vi "Send Message to Notebook.vi"(2 "Notebook Queue":refnum<queue>, 4 "Message":string, 5 "Error In":errorcluster, 9 "Text Formatting":T1={"Font"="Default", "Text Color"=enum."Unchanged", "Text Background Color"=enum."Unchanged", "Text Style"=enum."Regular", "Font Size (Points)"=-1.0, "Text Alignment"=0} {"Text Alignment" items=["Left", "Right", "Center"]}) -> (19 "Error Out":errorcluster)   [LabVIEW 2019, in "Notebook.lvlib"]
uses:
  Notebook.lvlib
  Notebook Action Q Element.ctl
  Notebook Action List.ctl
  Rich Text Box/Text Formatting.ctl
  Rich Text Box/Text Colors.ctl
  Rich Text Box/Formatted Text.ctl
  Rich Text Box/Rich Text Box.lvlib
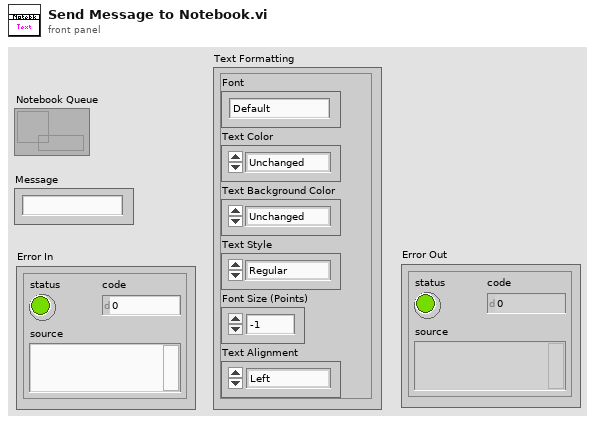
[diagram p1: front panel]
types:
  T1 = typedef "Rich Text Box.lvlib/Text Formatting.ctl" = cluster{"Font":string, "Text Color":T2, "Text Background Color":T2, "Text Style":enum16{"Regular", "Bold", "Italic", "Underline", "Strikeout"}, "Font Size (Points)":dbl, "Text Alignment":i32}
  T2 = typedef "Rich Text Box.lvlib/Text Colors.ctl" = enum16{"Unchanged", "Black", "Blue", "Brown", "Gray", "Green", "Orange", "Pink", "Red", "White"}
  T3 = typedef "Rich Text Box.lvlib/Formatted Text.ctl" = cluster{"Text":string, "Text Formatting":T1}
  T4 = typedef "Notebook.lvlib/Notebook Action Q Element.ctl" = cluster{"Action":T5, "Variant":variant}
  T5 = typedef "Notebook.lvlib/Notebook Action List.ctl" = enum16{"Idle", "Init", "Check Content Change", "User added content", "Program added text", "Program added Picture ", "Save Notebook", "Quit", "Open", "Close", "Update Window Title"}
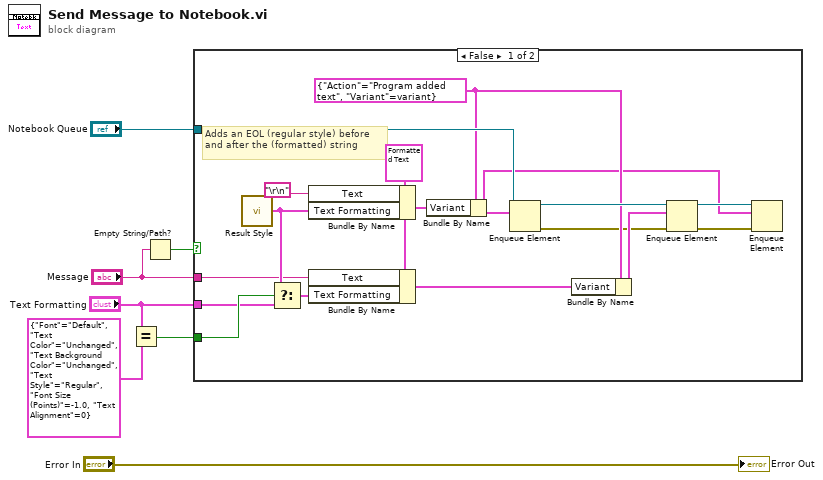
[diagram p0: block diagram]
diagram:
  n1 = Equal?(x="Text Formatting", y=T1 {"Font"="Default", "Text Color"=enum."Unchanged", "Text Background Color"=enum."Unchanged", "Text Style"=enum."Regular", "Font Size (Points)"=-1.0, "Text Alignment"=0} ("Text Formatting")) -> (x = y?=w6:bool)
  n2 = Empty String/Path?(string/path="Message") -> (empty?=w2:bool)
  n3 = case shown="False" w2 {
    tunnel: "Notebook Queue" -> [w23 _]
    tunnel: w6 -> [w12 _]
    tunnel: "Text Formatting" -> [w9 _]
    tunnel: "Message" -> [w8 _]
    frame False {
      w17 = T3 {"Text"="", "Text Formatting"={"Font"="Default", "Text Color"=enum."Unchanged", "Text Background Color"=enum."Unchanged", "Text Style"=enum."Regular", "Font Size (Points)"=-1.0, "Text Alignment"=0}} ("Formatted Text")
      w21 = T4 {"Action"=enum."Program added text", "Variant"=variant} ("element")
      # "Adds an EOL (regular style) before and after the (formatted) string"
      n4 = call "Result Style.vi"() -> ("Default Text Formatting"=w11:T1)
      n5 = Select(t=w11, s=w12, f=w9) -> (s? t:f=w10:T1)
      n6 = Bundle By Name(cluster=w17, "Text"="\r\n", "Text Formatting"=w11) -> (w19:T3)
      n7 = Bundle By Name(cluster=w17, "Text"=w8, "Text Formatting"=w10) -> (w13:T3)
      n8 = Bundle By Name(cluster=w21, "Variant"=w19) -> (w14:T4)
      n9 = Enqueue Element(queue=w23, element=w14) -> (queue out=w22:refnum<queue>, error out=w18:errorcluster)  [unwired: 2 in, 1 out]
      n10 = Bundle By Name(cluster=w21, "Variant"=w13) -> (w24:T4)
      n11 = Enqueue Element(queue=w22, element=w24, error in (no error)=w18) -> (queue out=w15:refnum<queue>, error out=w16:errorcluster)  [unwired: 1 in, 1 out]
      n12 = Enqueue Element(queue=w15, element=w14, error in (no error)=w16) -> ()  [unwired: 1 in, 3 out]
    }
    frame True {
    }
  }
  "Error Out" <- "Error In"
